vi "execute_quiry_command.vi"(2 "input_command":string, 3 "input_machine_reference.lvclass":refnum<class "machine.lvclass">) -> (0 "output_result":string, 1 "output_machine_reference.lvclass":refnum<class "machine.lvclass">)   [LabVIEW 2014, in "machine.lvclass"]
uses:
  machine.lvclass
  machine.lvclass/machine.ctl
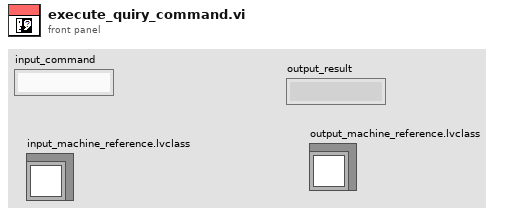
[diagram p1: front panel]
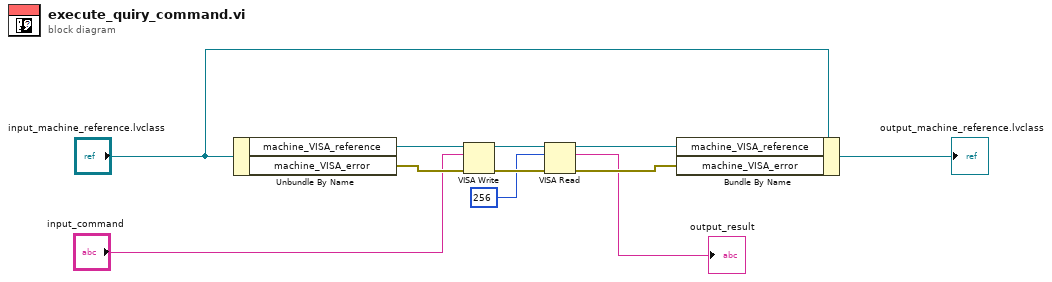
[diagram p0: block diagram]
diagram:
  n1 = Unbundle By Name("input_machine_reference.lvclass") -> ("machine_VISA_reference"=w11:refnum<visa-resource-name>, "machine_VISA_error"=w10:errorcluster)
  n2 = VISA Write(VISA resource name=w11, write buffer="input_command", error in (no error)=w10) -> (VISA resource name out=w6:refnum<visa-resource-name>, error out=w5:errorcluster)  [unwired: 1 out]
  n3 = VISA Read(VISA resource name=w6, byte count=u32 256, error in (no error)=w5) -> (VISA resource name out=w3:refnum<visa-resource-name>, read buffer=→"output_result":string, error out=w2:errorcluster)  [unwired: 1 out]
  n4 = Bundle By Name(cluster="input_machine_reference.lvclass", "machine_VISA_reference"=w3, "machine_VISA_error"=w2) -> (→"output_machine_reference.lvclass":refnum<class "machine.lvclass">)
